vi "Write Ramp Volt.vi"(8 "error in":errorcluster, 10 "Voltage_Ramp":dbl, 11 "69X_79X in":refnum<class "79XRP.lvclass">) -> (0 "error out":errorcluster, 3 "69X_79X out":refnum<class "79XRP.lvclass">)   [LabVIEW 2019, in "79XRP.lvlib" / "79XRP.lvclass"]
uses:
  Library/79XRP.lvclass
  builds/Instruments/PowerSupply.lvlibp/Library/PowerSupply.lvclass
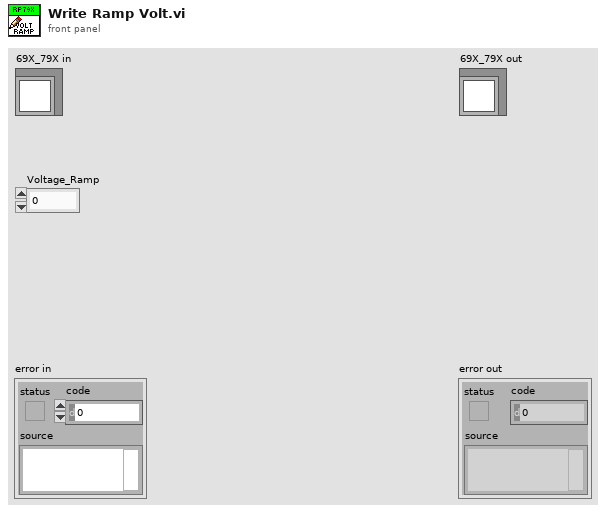
[diagram p1: front panel]
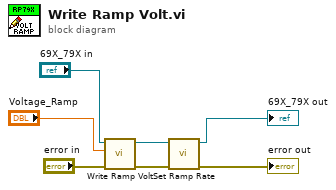
[diagram p0: block diagram]
diagram:
  n1 = call-parent "Write Ramp Volt.vi"("error in"="error in", "Voltage_Ramp"="Voltage_Ramp", "PowerSupply in"="69X_79X in") -> ("error out"=w4:errorcluster, "PowerSupply out"=w3:refnum<class "79XRP.lvclass">)  [unwired: 7 in]
  n2 = call "Set Ramp Rate.vi"("error in (no error)"=w4, "79XRP in"=w3) -> ("error out"=→"error out":errorcluster, "79XRP out"=→"69X_79X out":refnum<class "79XRP.lvclass">)  [unwired: 8 in]
